vi "Queues FGV.vi"(8 "error in":errorcluster, 11 "Action":T1) -> (0 "error out":errorcluster, 3 "Queues Out":T2)   [LabVIEW 2024, in "Tester InterComm.lvlib"]
uses:
  Tester InterComm.lvlib
  Process Queues.ctl
  QMH Item.ctl
  General Actions.ctl
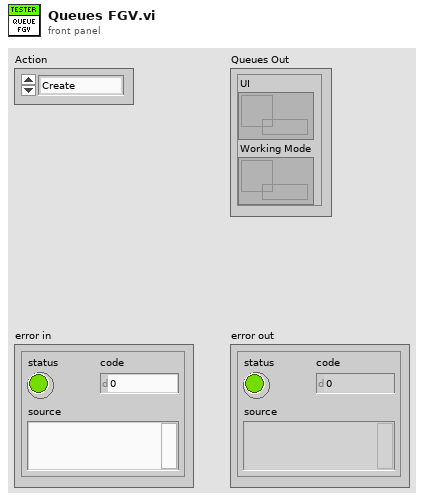
[diagram p1: front panel]
types:
  T1 = typedef "Tester InterComm.lvlib/General Actions.ctl" = enum16{"Create", "Get", "Destroy"}
  T2 = typedef "Tester InterComm.lvlib/Process Queues.ctl" = cluster{"UI":refnum<queue>, "Working Mode":refnum<queue>}
  T3 = typedef "Tester InterComm.lvlib/QMH Item.ctl" = cluster{"Message":string, "Data":variant}
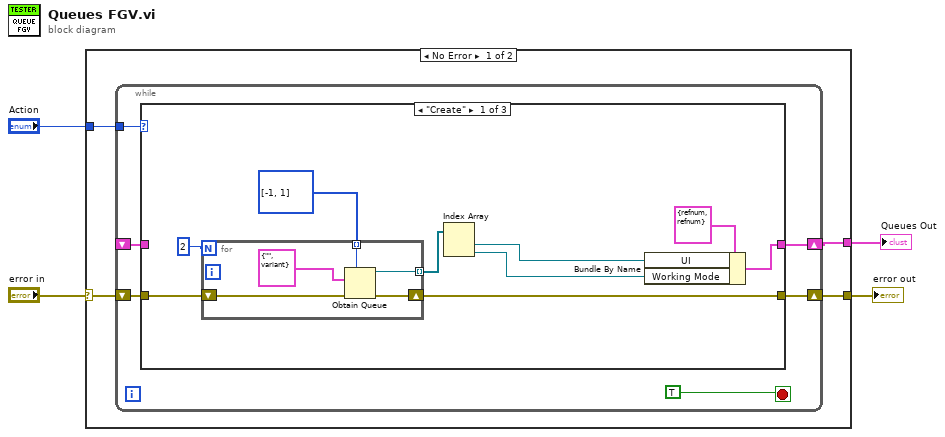
[diagram p0: block diagram]
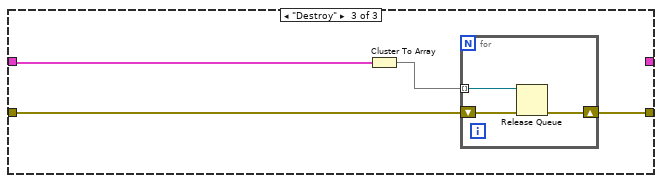
[diagram p3: hidden frame]
diagram:
  n1 = case shown="No Error" "error in" {
    selector: "error in" -> [w5 w38]
    tunnel: "Action" -> [w8 _]
    tunnel: [w7 w38] -> w3
    tunnel: [w6 _] -> w2
    frame No Error {
      n2 = while {
        tunnel: w8 -> [w13]
        shift-right: [w12] -> w7
        shift-left: w5 -> [w11]
        shift-right: [w10] -> w6
        shift-left: _ -> [w9]
        stop <- TRUE stop-if-true
        n3 = case shown="\"Create\"" w13 {
          tunnel: [w18 w30 w34] -> w12
          tunnel: w11 -> [w17 w30 w33]
          tunnel: [w22 w29 _] -> w10
          tunnel: w9 -> [_ w29 w31]
          frame "Create" {
            n4 = for {
              N: 2 -> [_]
              shift-right: [w27] -> w18
              shift-left: w17 -> [w28]
              tunnel: [w25] -> w21 mode=indexing
              tunnel: i32[] [-1, 1] -> [w24] mode=indexing
              n5 = Obtain Queue(max queue size (-1, unlimited)=w24, element data type=T3 {"Message"="", "Data"=variant}, error in (no error)=w28) -> (queue out=w25:refnum<queue>, error out=w27:errorcluster)  [unwired: 2 in, 1 out]
            }
            n6 = Index Array(array=w21) -> (element #1=w19:refnum<queue>, element #2=w16:refnum<queue>)  [unwired: 2 in]
            n7 = Bundle By Name(cluster=T2 {"UI"=refnum, "Working Mode"=refnum}, "UI"=w19, "Working Mode"=w16) -> (w22:T2)
          }
          frame "Get", Default {
          }
          frame "Destroy" {
            n8 = Cluster To Array(cluster=w31) -> (array=w32:refnum<queue>[])
            n9 = for {
              shift-right: [w36] -> w34
              shift-left: w33 -> [w37]
              tunnel: w32 -> [w35] mode=indexing
              n10 = Release Queue(queue=w35, error in (no error)=w37) -> (error out=w36:errorcluster)  [unwired: 1 in, 2 out]
            }
          }
        }
      }
    }
    frame Error {
    }
  }
  "error out" <- w3
  "Queues Out" <- w2
